vi "Convert Decimal to BCD.vi"(4 "Frequency, 10xMHz":u32 format="%.0b") -> (1 "BCD Frequency":u32 format="%.0b")   [LabVIEW 2011]
doc: "Accepts an unsigned, 32 bit decimal value and returns an unsigned, 32 bit integer representing the BCD coded decimal value. In BCD, each decimal digit is broken down into a 4-bit representation."
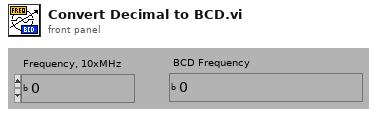
[diagram p1: front panel]
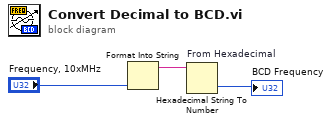
[diagram p0: block diagram]
diagram:
  n1 = Format Into String "Format Into String"("Frequency, 10xMHz") -> (resulting string=w1:string)  [unwired: 3 in, 1 out]
  n2 = Hexadecimal String To Number "From Hexadecimal"(string=w1) -> (number=→"BCD Frequency":u32)  [unwired: 3 out]
